vi "Build Array.vi"(10 "value":dbl) -> (2 "Array":dbl[](array[numeric]))   [LabVIEW 2021]
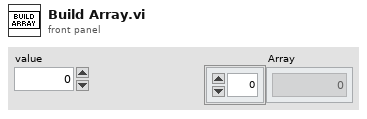
[diagram p1: front panel]
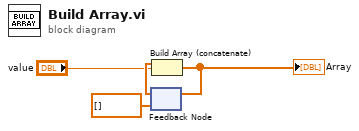
[diagram p0: block diagram]
diagram:
  n1 = feedback #1(dbl[] []) -> (w4:dbl[])
  n2 = Build Array (concatenate)(w4, "value") -> (w3:dbl[])
  "Array" <- w3
  n3 = feedback-in #1(w3) -> ()
